vi "UI Initialize.vi"(8 "error in (no error)":errorcluster, 11 "GObject View in":refnum<class "VI List View.lvclass">) -> (0 "error out":errorcluster, 3 "GObject View out":refnum<class "VI List View.lvclass">)   [LabVIEW 2013, in "SET Project Editor.lvlib" / "VI List View.lvclass"]
uses:
  VI List View.lvclass
  <vilib>/Utility/miscctls.llb/LVRowAndColumnTypeDef.ctl
  UI View/UI View.lvclass
  VI List View.lvclass/VI List View.ctl
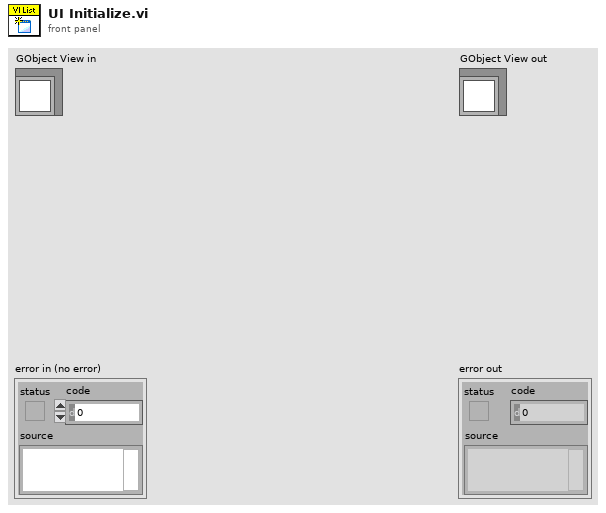
[diagram p1: front panel]
types:
  T1 = typedef "LVRowAndColumnTypeDef.ctl" = cluster{"Row":i32, "Column":i32}
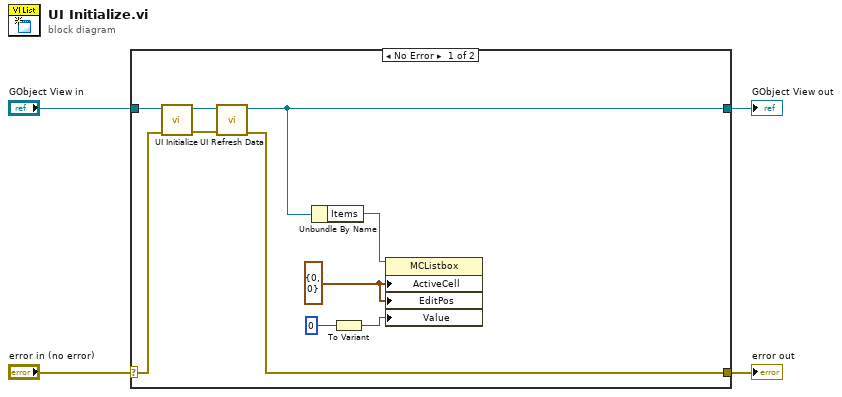
[diagram p0: block diagram]
diagram:
  n1 = case shown="No Error" "error in (no error)" {
    selector: "error in (no error)" -> [w8 w16]
    tunnel: [w10 w16] -> w3
    tunnel: [w5 w15] -> w1
    tunnel: "GObject View in" -> [w9 w15]
    frame No Error {
      w11 = T1 {"Row"=0, "Column"=0} ("Active Cell:Active Cell")
      n2 = call-parent "UI Initialize.vi"("error in (no error)"=w8, "UI View in"=w9) -> ("error out"=w7:errorcluster, "UI View out"=w6:refnum<class "VI List View.lvclass">)  [unwired: 8 in]
      n3 = call-dynamic "UI Refresh Data.vi"("error in (no error)"=w7, "GObject View in"=w6) -> ("error out"=w10:errorcluster, "GObject View out"=w5:refnum<class "VI List View.lvclass">)  [unwired: 8 in]
      n4 = Unbundle By Name(w5) -> ("Items"=w14:refnum<vi>)
      n5 = To Variant(anything=0) -> (Variant=w12:variant)
      n6 = property class="MCListbox"(reference=w14, "ActiveCell"=w11, "EditPos"=w11, "Value"=w12) -> ()  [unwired: 1 in, 2 out]
    }
    frame Error {
    }
  }
  "error out" <- w3
  "GObject View out" <- w1
